vi "extremeOfNinePixel.vi"(0 "4":i8, 1 "3":i8, 2 "2":i8, 3 "1":i8, 7 "5":i8, 11 "6":i8, 12 "7":i8, 13 "8":i8, 14 "9":i8, 15 "extreme Type":u8) -> (6 "extreme out":i8)   [LabVIEW 2016]
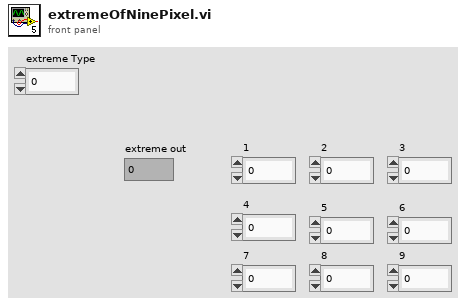
[diagram p1: front panel]
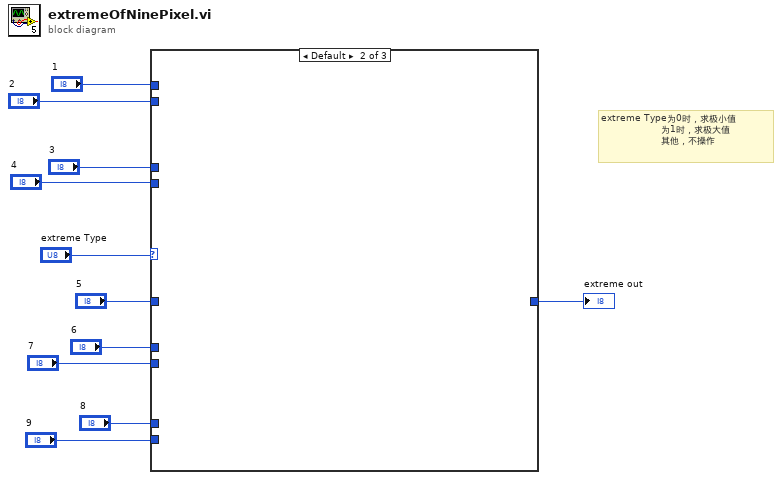
[diagram p0: block diagram]
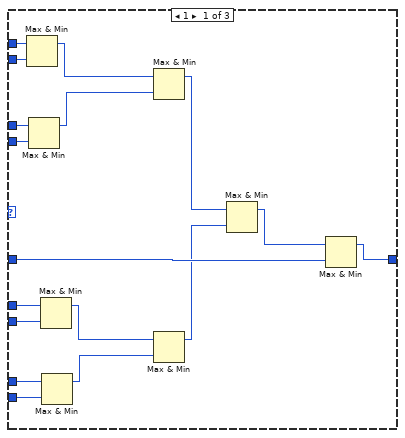
[diagram p2: hidden frame]
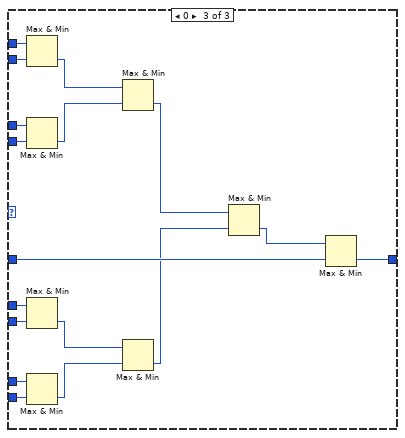
[diagram p3: hidden frame]
diagram:
  # "extreme Type为0时，求极小值\n                    为1时，求极大值\n                    其他，不操作"
  n1 = case shown="Default" "extreme Type" {
    tunnel: "1" -> [w28 _ w45]
    tunnel: "2" -> [w27 _ w44]
    tunnel: "3" -> [w26 _ w43]
    tunnel: "4" -> [w25 _ w42]
    tunnel: "8" -> [w24 _ w41]
    tunnel: "9" -> [w23 _ w40]
    tunnel: "7" -> [w22 _ w39]
    tunnel: "6" -> [w21 _ w38]
    tunnel: "5" -> [w16 _ w37]
    tunnel: [w15 _ w29] -> w11
    frame 1 {
      n2 = Max & Min(x=w28, y=w27) -> (max(x,y)=w20:i8)  [unwired: 1 out]
      n3 = Max & Min(x=w26, y=w25) -> (max(x,y)=w19:i8)  [unwired: 1 out]
      n4 = Max & Min(x=w21, y=w22) -> (max(x,y)=w18:i8)  [unwired: 1 out]
      n5 = Max & Min(x=w24, y=w23) -> (max(x,y)=w17:i8)  [unwired: 1 out]
      n6 = Max & Min(x=w20, y=w19) -> (max(x,y)=w14:i8)  [unwired: 1 out]
      n7 = Max & Min(x=w18, y=w17) -> (max(x,y)=w13:i8)  [unwired: 1 out]
      n8 = Max & Min(x=w14, y=w13) -> (max(x,y)=w12:i8)  [unwired: 1 out]
      n9 = Max & Min(x=w12, y=w16) -> (max(x,y)=w15:i8)  [unwired: 1 out]
    }
    frame Default {
    }
    frame 0 {
      n10 = Max & Min(x=w45, y=w44) -> (min(x,y)=w36:i8)  [unwired: 1 out]
      n11 = Max & Min(x=w43, y=w42) -> (min(x,y)=w35:i8)  [unwired: 1 out]
      n12 = Max & Min(x=w38, y=w39) -> (min(x,y)=w34:i8)  [unwired: 1 out]
      n13 = Max & Min(x=w41, y=w40) -> (min(x,y)=w33:i8)  [unwired: 1 out]
      n14 = Max & Min(x=w36, y=w35) -> (min(x,y)=w31:i8)  [unwired: 1 out]
      n15 = Max & Min(x=w34, y=w33) -> (min(x,y)=w32:i8)  [unwired: 1 out]
      n16 = Max & Min(x=w31, y=w32) -> (min(x,y)=w30:i8)  [unwired: 1 out]
      n17 = Max & Min(x=w30, y=w37) -> (min(x,y)=w29:i8)  [unwired: 1 out]
    }
  }
  "extreme out" <- w11
